vi "DeserializeParameters.vi"(8 "error in (no error)":errorcluster, 10 "Variant":variant, 11 "BananaPeel in":refnum<class "BananaPeel.lvclass">) -> (0 "error out":errorcluster, 3 "BananaPeel out":refnum<class "BananaPeel.lvclass">)   [LabVIEW 2021, in "Bananas.lvlib" / "BananaPeel.lvclass"]
uses:
  BananaPeel.lvclass
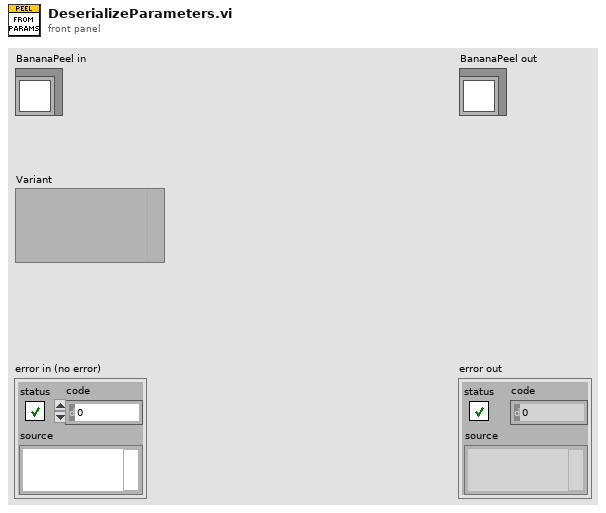
[diagram p1: front panel]
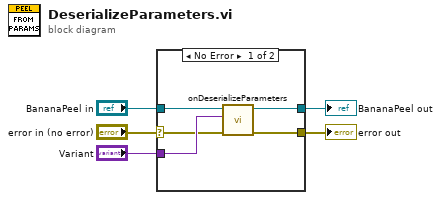
[diagram p0: block diagram]
diagram:
  n1 = case shown="No Error" "error in (no error)" {
    selector: "error in (no error)" -> [w7 w12]
    tunnel: [w6 w12] -> w4
    tunnel: [w10 w11] -> w2
    tunnel: "BananaPeel in" -> [w9 w11]
    tunnel: "Variant" -> [w8 _]
    frame No Error {
      n2 = call-dynamic "onDeserializeParameters.vi"("error in (no error)"=w7, "Variant"=w8, "BananaPeel in"=w9) -> ("error out"=w6:errorcluster, "BananaPeel out"=w10:refnum<class "BananaPeel.lvclass">)  [unwired: 7 in]
    }
    frame Error {
    }
  }
  "error out" <- w4
  "BananaPeel out" <- w2
